vi "Write-out Google Maps.vi"(0 "Latitude":string, 2 "Longitude":string) -> (6 "KML Data":string)   [LabVIEW 2015]
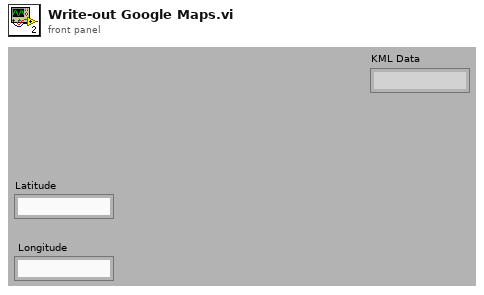
[diagram p1: front panel]
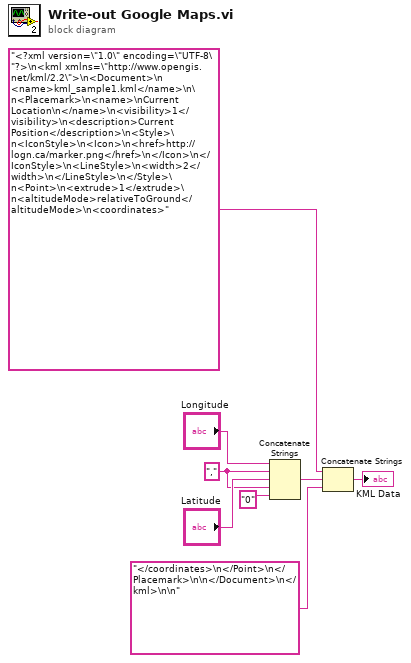
[diagram p0: block diagram]
diagram:
  w3 = ","
  n1 = Concatenate Strings("Longitude", w3, "Latitude", w3, "0" ("string")) -> (w4:string)
  n2 = Concatenate Strings("<?xml version=\"1.0\" encoding=\"UTF-8\"?>\n<kml xmlns=\"http://www.opengis.net/kml/2.2\">\n<Document>\n  <name>kml_sample1.kml</name>\n\n<Placemark>\n<name>\nCurrent Location\n</name>\n<visibility>1</visibility>\n<description>Current Position</description>\n<Style>\n<IconStyle>\n<Icon>\n<href>http://logn.ca/marker.png</href>\n</Icon>\n</IconStyle>\n<LineStyle>\n<width>2</width>\n</LineStyle>\n</Style>\n<Point>\n<extrude>1</extrude>\n<altitudeMode>relativeToGround</altitudeMode>\n<coordinates>", w4, "</coordinates>\n</Point>\n</Placemark>\n\n</Document>\n</kml>\n\n") -> (→"KML Data":string)
